vi "Launcher - Head Worker.vi"(6 "Worker Alias":string="cRIO Head Worker", 8 "error in":errorcluster, 9 "Initialization Data":T1={"Client Name"="cRIO TCP Client", "Server IP Address"="", "Server Port"=9123}, 11 "Head Worker in":refnum<class "Head Worker.lvclass">) -> (0 "error out":errorcluster)   [LabVIEW 2017]
doc: "This VI launches the Head Worker of a Workers application."
uses:
  Workers/Head Worker/Initialization Data.ctl
  Workers/Head Worker/Head Worker.lvclass
  C:/Program Files (x86)/National Instruments/LabVIEW 2017/vi.lib/addons/_Workers/Library/Classes/Worker/Worker.lvclass
  <vilib>/addons/_Workers/Debugger/Debug Client/Debug Client.lvlib
panel:
  # "<- Change here the IP address of the Host PC"
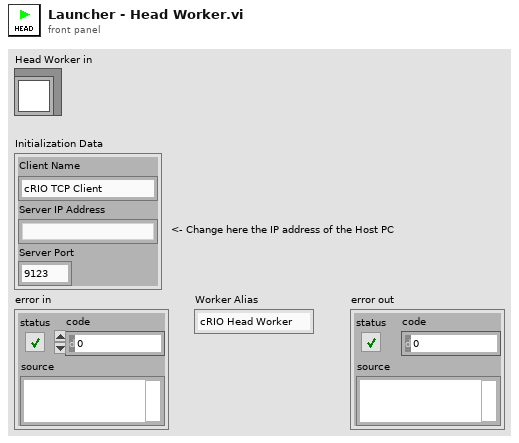
[diagram p1: front panel]
types:
  T1 = typedef "Head Worker.lvclass/Initialization Data.ctl" = cluster{"Client Name":string, "Server IP Address":string, "Server Port":u16}
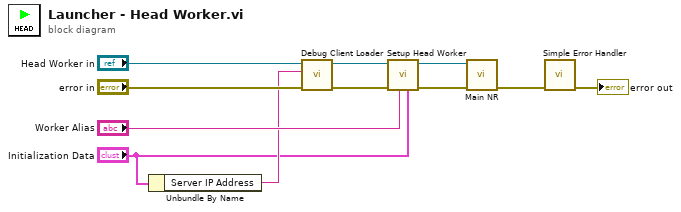
[diagram p0: block diagram]
diagram:
  n1 = Unbundle By Name("Initialization Data") -> ("Server IP Address"=w2:string)
  n2 = call <vilib>:"Debug Client Loader.vi"("error in (no error)"="error in", "Debug Server IP Address (127.0.0.1)"=w2, "Worker_"="Head Worker in") -> ("error out"=w5:errorcluster, "Worker_out"=w3:refnum<class "Head Worker.lvclass">)  [unwired: 7 in]
  n3 = call-dynamic "Setup Head Worker.vi"("Initalization Data"="Initialization Data", "Worker Alias"="Worker Alias", "error in"=w5, "Worker_"=w3) -> ("error out"=w11:errorcluster, "Worker_out"=w8:refnum<class "Head Worker.lvclass">)  [unwired: 6 in]
  n4 = call-dynamic "Main NR.vi"("error in"=w11, "Head Worker in"=w8) -> ("error out"=w9:errorcluster)  [unwired: 8 in, 1 out]
  n5 = call <vilib>:"Simple Error Handler.vi"("error in (no error)"=w9) -> ("error out"=→"error out":errorcluster)  [unwired: 4 in, 4 out]
